vi "deeplabv3_postprocess.vi"(6 "colors":u32[](array[numeric]), 8 "error in (no error)":errorcluster, 9 "1d_data":sgl[](array[numeric]), 10 "length":i32[](array[numeric]), 11 "img in":refnum<class "Mat_8U.lvclass">) -> (0 "error out":errorcluster, 2 "mask":refnum<class "Mat_8U.lvclass">, 3 "img out":refnum<class "Mat_8U.lvclass">)   [LabVIEW 2018]
uses:
  <vilib>/addons/VIRobotics/opencv_yiku/Mat/Mat_8U/Mat_8U.lvclass
  C:/Program Files/National Instruments/LabVIEW 2018_64bit/vi.lib/addons/VIRobotics/opencv_yiku/Mat/Mat/Mat.lvclass
  <vilib>/addons/VIRobotics/opencv_yiku/Mat/Create_Mat_8U.vi
  <vilib>/addons/VIRobotics/opencv_yiku/opencv_yiku.lvlib
panel:
  out "error out 4":errorcluster
  out "error out 3":errorcluster
  out "error out 2":errorcluster
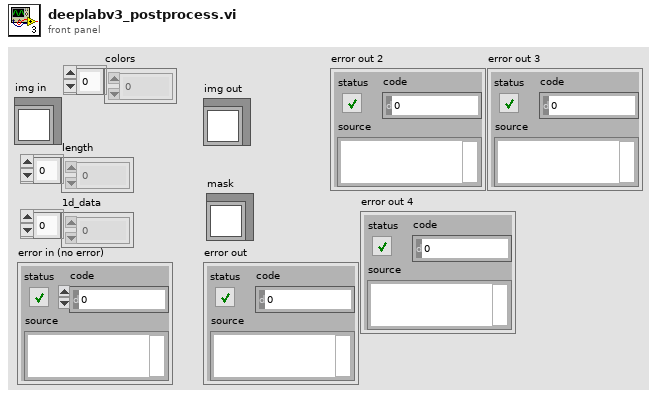
[diagram p1: front panel]
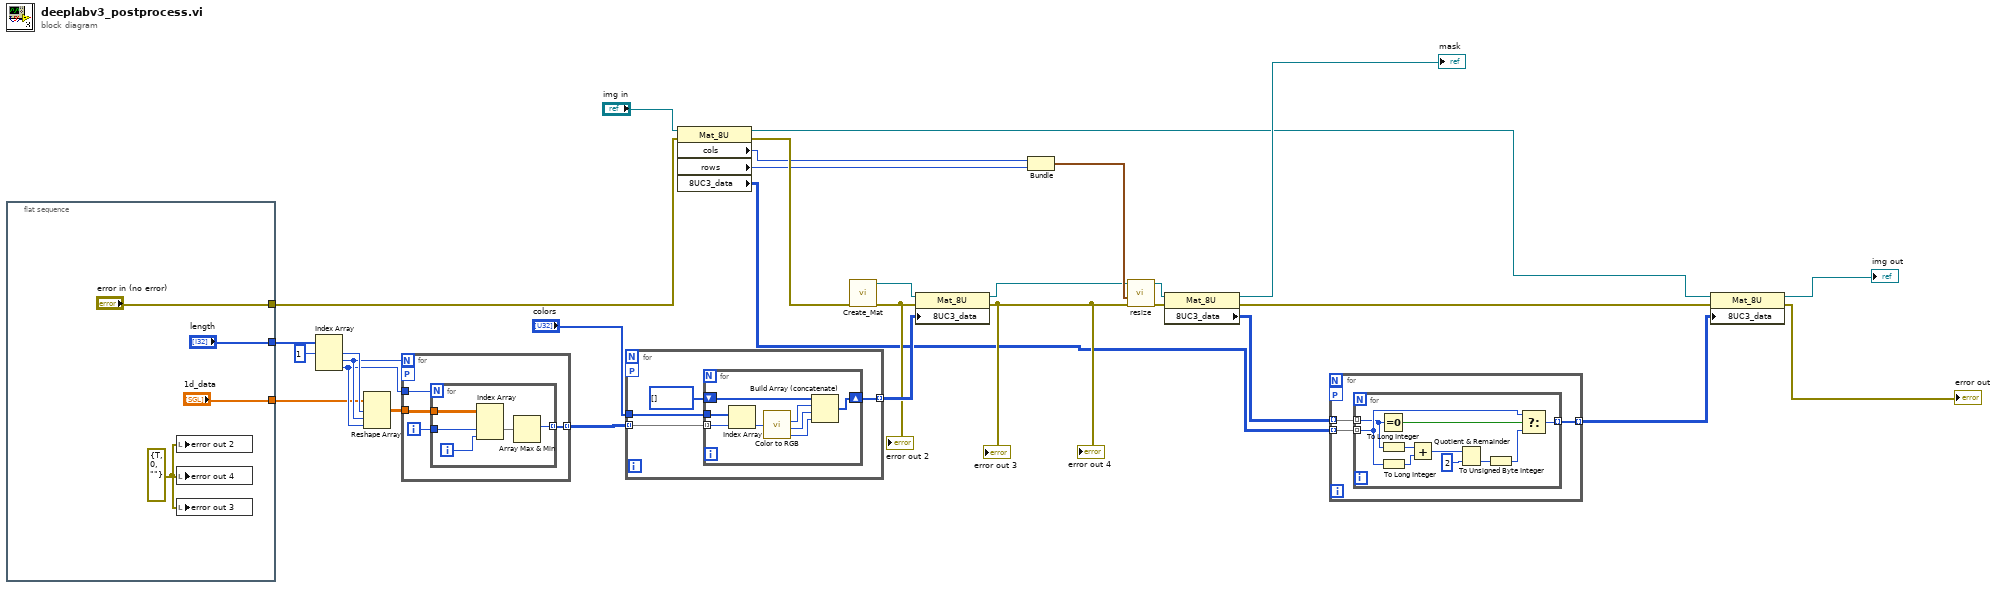
[diagram p0: block diagram]
diagram:
  n1 = flat-sequence {
    tunnel: ["1d_data"] -> w11
    tunnel: ["length"] -> w10
    tunnel: ["error in (no error)"] -> w8
    frame #0 {
      w31 = errorcluster {"status"=TRUE, "code"=0, "source"=""} ("error out 3")
      n2 = local write "error out 2"(w31) -> ()
      n3 = local write "error out 4"(w31) -> ()
      n4 = local write "error out 3"(w31) -> ()
    }
  }
  n5 = Index Array(array=w10, index #1=1 ("index")) -> (element #1=w23:i32, element #2=w22:i32, element #3=w21:i32)  [unwired: 2 in]
  n6 = Reshape Array(w11, w23, w22, w21) -> (w15:sgl[][][])
  n7 = for {
    N: w22 -> [_]
    tunnel: w15 -> [w38]
    tunnel: w21 -> [w36]
    tunnel: [w35] -> w16 mode=indexing
    workers-P: _ -> [_]
    i -> [w37]
    n8 = for {
      N: w36 -> [_]
      tunnel: w38 -> [w43]
      tunnel: w37 -> [w42]
      tunnel: [w39] -> w35 mode=indexing
      i -> [w41]
      n9 = Index Array(array=w43, index (dim 1)=w42, index (dim 2)=w41) -> (element=w40:sgl[])  [unwired: 1 in]
      n10 = Array Max & Min(array=w40) -> (max index (indices)=w39:i32)  [unwired: 3 out]
    }
  }
  n11 = for {
    tunnel: w16 -> [w47] mode=indexing
    tunnel: "colors" -> [w46]
    tunnel: [w44] -> w25 mode=indexing
    workers-P: _ -> [_]
    n12 = for {
      tunnel: w47 -> [w54] mode=indexing
      tunnel: w46 -> [w55]
      shift-right: [w48] -> w44
      shift-left: u8[] [] -> [w53]
      n13 = Index Array(array=w55, index=w54) -> (element=w52:u32)
      n14 = call <vilib>:"Color to RGB.vi"("Color"=w52) -> ("R"=w51:u8, "G"=w50:u8, "B"=w49:u8)  [unwired: 1 out]
      n15 = Build Array (concatenate)(w53, w51, w50, w49) -> (w48:u8[])
    }
  }
  n16 = property class="Mat_8U"(reference="img in", error in=w8) -> (reference out=w5:refnum<class "Mat_8U.lvclass">, error out=w7:errorcluster, "cols"=w3:i32, "rows"=w2:i32, "8UC3_data"=w4:u8[][])
  n17 = call-poly <vilib>:"Create_Mat.vi"("error in (no error)"=w7) -> ("error out"=w19:errorcluster, "Mat_8U_out"=w24:refnum<class "Mat_8U.lvclass">)  [unwired: 9 in]
  "error out 2" <- w19
  n18 = property class="Mat_8U"(reference=w24, error in=w19, "8UC3_data"=w25) -> (reference out=w26:refnum<class "Mat_8U.lvclass">, error out=w6:errorcluster)
  "error out 3" <- w6
  "error out 4" <- w6
  n19 = Bundle("cols"=w3, "rows"=w2) -> (w27:cluster{"cols":i32, "rows":i32})  [unwired: 1 in]
  n20 = call <vilib>:"resize.vi"("error in (no error)"=w6, "Size"=w27, "src"=w26) -> ("error out"=w18:errorcluster, "src out"=w28:refnum<class "Mat_8U.lvclass">)  [unwired: 6 in, 1 out]
  n21 = property class="Mat_8U"(reference=w28, error in=w18) -> (reference out=→"mask":refnum<class "Mat_8U.lvclass">, error out=w17:errorcluster, "8UC3_data"=w29:u8[][])
  n22 = for {
    tunnel: w29 -> [w58] mode=indexing
    tunnel: w4 -> [w57] mode=indexing
    tunnel: [w56] -> w12 mode=indexing
    workers-P: _ -> [_]
    n23 = for {
      tunnel: w58 -> [w59] mode=indexing
      tunnel: w57 -> [w64] mode=indexing
      tunnel: [w65] -> w56 mode=indexing
      n24 = Equal To 0?(x=w59) -> (x = 0?=w68:bool)
      n25 = To Long Integer(number=w59) -> (32bit integer=w62:i32)
      n26 = To Long Integer(number=w64) -> (32bit integer=w63:i32)
      n27 = Add(x=w62, y=w63) -> (x+y=w67:i32)
      n28 = Quotient & Remainder(x=w67, y=u8 2) -> (floor(x/y)=w61:i32)  [unwired: 1 out]
      n29 = To Unsigned Byte Integer(number=w61) -> (unsigned 8bit integer=w60:u8)
      n30 = Select(t=w64, s=w68, f=w60) -> (s? t:f=w65:u8)
    }
  }
  n31 = property class="Mat_8U"(reference=w5, error in=w17, "8UC3_data"=w12) -> (reference out=→"img out":refnum<class "Mat_8U.lvclass">, error out=→"error out":errorcluster)
